vi "Write Board.vi"(10 "Board":refnum<class "Board.lvclass">, 11 "Position in":refnum<class "Position.lvclass">) -> (3 "Position out":refnum<class "Position.lvclass">)   [LabVIEW 2016, in "Chesslib.lvlib" / "Position.lvclass"]
uses:
  Position.lvclass
  Board/Board.lvclass
  Position.lvclass/Position.ctl
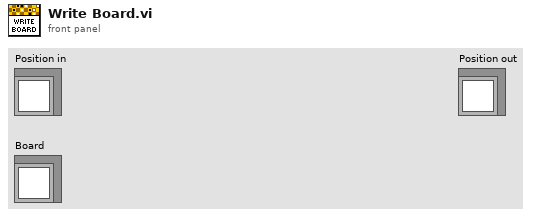
[diagram p1: front panel]
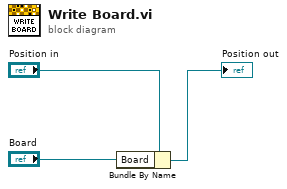
[diagram p0: block diagram]
diagram:
  n1 = Bundle By Name(cluster="Position in", "Board"="Board") -> (→"Position out":refnum<class "Position.lvclass">)
